vi "Configure Measurement.vi"(5 "Enable Gate Feed (T: Enable)":bool=TRUE, 6 "Measurement Function (0: Average)":i32(ring) items=["Average", "Normal"], 7 "Measurement Rate (0: Normal)":i32(ring) items=["Normal", "Double", "Fast"], 8 "error in (no error)":errorcluster, 9 "Resolution (1)":dbl=1.0, 10 "Expected Value (0)":dbl, 11 "VISA resource name":refnum<visa-resource-name>) -> (0 "error out":errorcluster, 3 "VISA resource name out":refnum<visa-resource-name>)   [LabVIEW 2018, in "Agilent U2000 Series.lvlib"]
doc: "Configures the instrument to take single or dual channel measurements.\n\nNote:\nThis VI is not applicable for Agilent U2021/2XA. Please use <B>Configure Measurement Characteristic.vi</B> instead."
uses:
  Agilent U2000 Series.lvlib
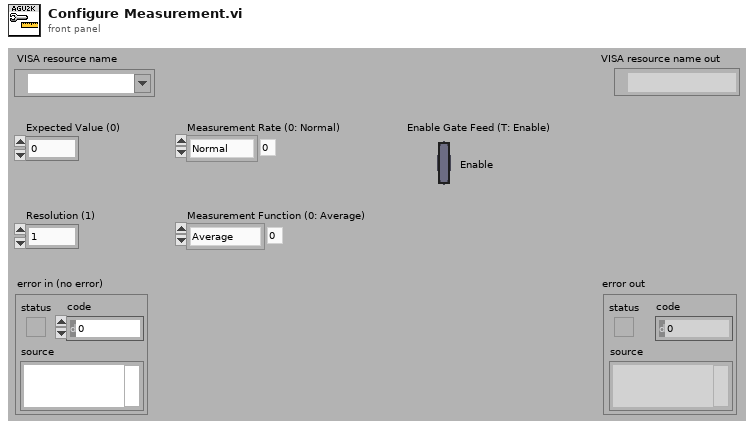
[diagram p1: front panel]
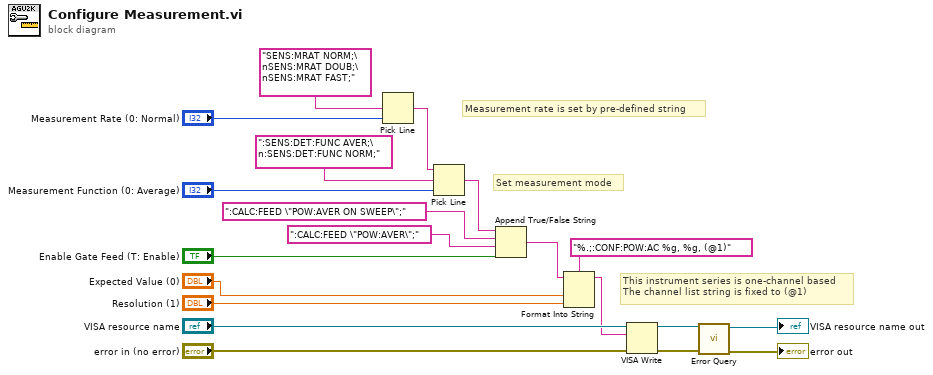
[diagram p0: block diagram]
diagram:
  # "This instrument series is one-channel based\nThe channel list string is fixed to (@1)"
  # "Set measurement mode"
  # "Measurement rate is set by pre-defined string"
  n1 = Pick Line(multi-line string="SENS:MRAT NORM;\nSENS:MRAT DOUB;\nSENS:MRAT FAST;", line index="Measurement Rate (0: Normal)") -> (output string=w16:string)  [unwired: 1 out]
  n2 = Pick Line(string ("")=w16, multi-line string=":SENS:DET:FUNC AVER;\n:SENS:DET:FUNC NORM;", line index="Measurement Function (0: Average)") -> (output string=w15:string)
  n3 = Append True/False String(1:"Enable Gate Feed (T: Enable)", 2:":CALC:FEED \"POW:AVER\";", 3:":CALC:FEED \"POW:AVER ON SWEEP\";", 4:w15) -> (0:w6:string)
  n4 = Format Into String(format string="%.;:CONF:POW:AC %g, %g, (@1)", initial string=w6, "Expected Value (0)", "Resolution (1)") -> (resulting string=w5:string)  [unwired: 1 in, 1 out]
  n5 = VISA Write(VISA resource name="VISA resource name", write buffer=w5, error in (no error)="error in (no error)") -> (VISA resource name out=w4:refnum<visa-resource-name>, error out=w3:errorcluster)  [unwired: 1 out]
  n6 = call "Error Query.vi"("error in (no error)"=w3, "VISA resource name"=w4) -> ("error out"=→"error out":errorcluster, "VISA resource name out"=→"VISA resource name out":refnum<visa-resource-name>)  [unwired: 8 out]
